vi "Table 2 Structure.vi"(10 "Table Control":string[][](table)=[["Patient Number", "057235558", ""], ["Eye", "Right Eye", ""], ["Treatment Area", "Full 360", ""], ["Eye Color", "Blue/Green", ""], ["Avg. Pulse Energy", "1.4mJ", ""], ["Number of Pulses", "100", ""], ["Time Between Pulses", "8.0mSec", ""], ["Distance from Limbus", "200.0um", ""], ["Illumination Intensity", "12", ""], ["Aiming Beam Intensity", "5", ""], ["Raneging Beam Intensity", "5", ""]]) -> (2 "Eagle Data":T1)   [LabVIEW 2015]
uses:
  Controls/Eagle Data.ctl
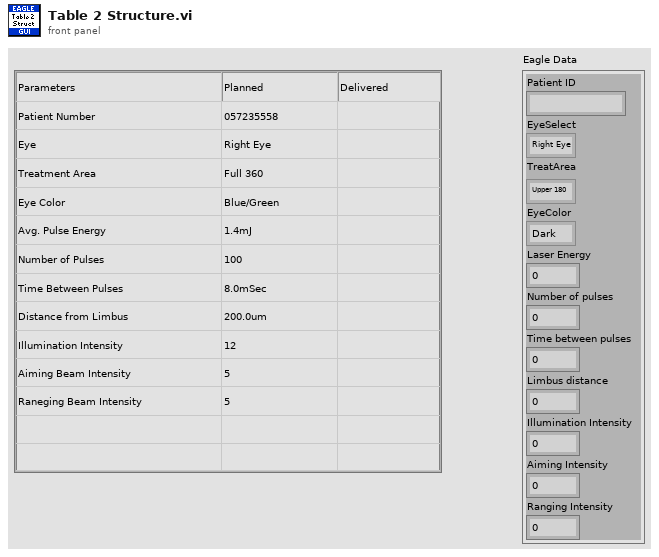
[diagram p1: front panel]
types:
  T1 = typedef "Eagle Data.ctl" = cluster{"Patient ID":string, "EyeSelect":enum32{"Right Eye", "Left Eye"}, "TreatArea":enum32{"Upper 180", "Lower 180", "Full 360"}, "EyeColor":enum32{"Dark", "Blue/Green"}, "Laser Energy":dbl, "Number of pulses":u8, "Time between pulses":dbl, "Limbus distance":dbl, "Illumination Intensity":dbl, "Aiming Intensity":dbl, "Ranging Intensity":dbl}
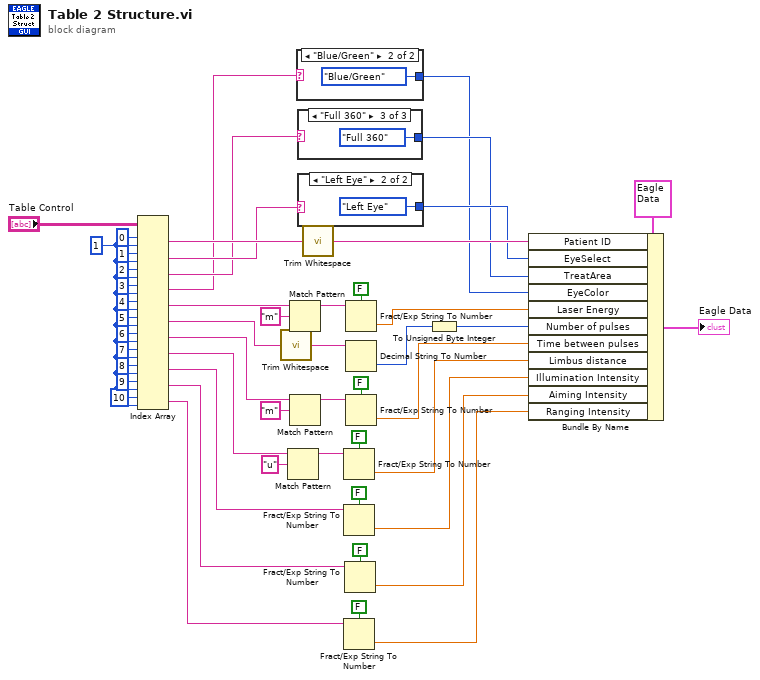
[diagram p0: block diagram]
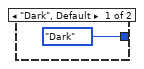
[diagram p2: hidden frame]
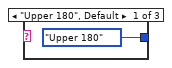
[diagram p3: hidden frame]
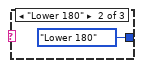
[diagram p4: hidden frame]
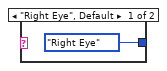
[diagram p5: hidden frame]
diagram:
  w50 = 1 ("disabled index (col)")
  n1 = Index Array(array="Table Control", index (row) #1=0 ("disabled index (row)"), index (col) #1=w50, index (row) #2=1 ("disabled index (row)"), index (col) #2=w50, index (row) #3=2 ("disabled index (row)"), index (col) #3=w50, index (row) #4=3 ("disabled index (row)"), index (col) #4=w50, index (row) #5=4 ("disabled index (row)"), index (col) #5=w50, index (row) #6=5 ("disabled index (row)"), index (col) #6=w50, index (row) #7=6 ("disabled index (row)"), index (col) #7=w50, index (row) #8=7 ("disabled index (row)"), index (col) #8=w50, index (row) #9=8 ("disabled index (row)"), index (col) #9=w50, index (row) #10=9 ("disabled index (row)"), index (col) #10=w50, index (row) #11=10 ("disabled index (row)"), index (col) #11=w50) -> (element #1=w36:string, element #2=w34:string, element #3=w32:string, element #4=w30:string, element #5=w28:string, element #6=w23:string, element #7=w16:string, element #8=w11:string, element #9=w6:string, element #10=w4:string, element #11=w1:string)
  n2 = call <vilib>:"Trim Whitespace.vi"("string"=w23) -> ("trimmed string"=w22:string)  [unwired: 1 in]
  n3 = Match Pattern(string=w11, regular expression="u") -> (before substring=w13:string)  [unwired: 1 in, 3 out]
  n4 = Match Pattern(string=w28, regular expression="m") -> (before substring=w26:string)  [unwired: 1 in, 3 out]
  n5 = Match Pattern(string=w16, regular expression="m") -> (before substring=w18:string)  [unwired: 1 in, 3 out]
  n6 = case shown="\"Blue/Green\"" w30 {
    tunnel: [enum32{"Dark", "Blue/Green"}."Dark" ("EyeColor") enum32{"Dark", "Blue/Green"}."Blue/Green" ("EyeColor")] -> w29
    frame "Dark", Default {
    }
    frame "Blue/Green" {
    }
  }
  n7 = case shown="\"Full 360\"" w32 {
    tunnel: [enum32{"Upper 180", "Lower 180", "Full 360"}."Upper 180" ("TreatArea") enum32{"Upper 180", "Lower 180", "Full 360"}."Lower 180" ("TreatArea") enum32{"Upper 180", "Lower 180", "Full 360"}."Full 360" ("TreatArea")] -> w31
    frame "Upper 180", Default {
    }
    frame "Lower 180" {
    }
    frame "Full 360" {
    }
  }
  n8 = case shown="\"Left Eye\"" w34 {
    tunnel: [enum32{"Right Eye", "Left Eye"}."Right Eye" ("EyeSelect") enum32{"Right Eye", "Left Eye"}."Left Eye" ("EyeSelect")] -> w33
    frame "Right Eye", Default {
    }
    frame "Left Eye" {
    }
  }
  n9 = call <vilib>:"Trim Whitespace.vi"("string"=w36) -> ("trimmed string"=w35:string)  [unwired: 1 in]
  n10 = Fract/Exp String To Number(use system decimal point (T)=FALSE, string=w13) -> (number=w10:dbl)  [unwired: 2 in, 1 out]
  n11 = Fract/Exp String To Number(use system decimal point (T)=FALSE, string=w6) -> (number=w5:dbl)  [unwired: 2 in, 1 out]
  n12 = Fract/Exp String To Number(use system decimal point (T)=FALSE, string=w1) -> (number=w2:dbl)  [unwired: 2 in, 1 out]
  n13 = Fract/Exp String To Number(use system decimal point (T)=FALSE, string=w4) -> (number=w3:dbl)  [unwired: 2 in, 1 out]
  n14 = Fract/Exp String To Number(use system decimal point (T)=FALSE, string=w26) -> (number=w24:dbl)  [unwired: 2 in, 1 out]
  n15 = Decimal String To Number(string=w22) -> (number=w21:i32)  [unwired: 2 in, 1 out]
  n16 = Fract/Exp String To Number(use system decimal point (T)=FALSE, string=w18) -> (number=w15:dbl)  [unwired: 2 in, 1 out]
  n17 = To Unsigned Byte Integer(number=w21) -> (unsigned 8bit integer=w20:u8)
  n18 = Bundle By Name(cluster=T1 {"Patient ID"="", "EyeSelect"=enum."Right Eye", "TreatArea"=enum."Upper 180", "EyeColor"=enum."Dark", "Laser Energy"=0.0, "Number of pulses"=0, "Time between pulses"=0.0, "Limbus distance"=0.0, "Illumination Intensity"=0.0, "Aiming Intensity"=0.0, "Ranging Intensity"=0.0} ("Eagle Data"), "Patient ID"=w35, "EyeSelect"=w33, "TreatArea"=w31, "EyeColor"=w29, "Laser Energy"=w24, "Number of pulses"=w20, "Time between pulses"=w15, "Limbus distance"=w10, "Illumination Intensity"=w5, "Aiming Intensity"=w3, "Ranging Intensity"=w2) -> (→"Eagle Data":T1)
